vi "Main.vi"() -> ()   [LabVIEW 2012]
panel:
  out "x+1":dbl
  out "x+y":dbl
  in  "y":dbl
  in  "x":dbl
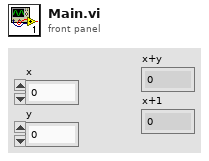
[diagram p1: front panel]
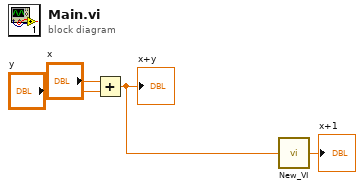
[diagram p0: block diagram]
diagram:
  n1 = Add(x="x", y="y") -> (x+y=w2:dbl)
  "x+y" <- w2
  n2 = call "New_VI.vi"("Numeric"=w2) -> ("x+1"=→"x+1":dbl)
